vi "Stop cameras.vi"(4 "MASTER in":T1 {"Image data"."Color Palette" items=["Grayscale U8", "False Color", "Overexposed"]; "Image data"."Exposure time [us]" format="%#_10g"; "Queue"."Initial time [s]" format="%_19f"; "Queue"."Raw data [V]\n(all samples)" format="%0.2f"; "Queue"."Timestamp [s]" format="%_19f"}) -> ()   [LabVIEW 2020]
uses:
  MASTER.ctl
  Constants.ctl
  QBundle.ctl
  Queue.ctl
  Image data.ctl
  <vilib>/userdefined/High Color/IMAQdx.ctl
  <vilib>/vision/Image Controls.llb/IMAQ Image.ctl
  Image QBundle.ctl
  <vilib>/vision/driver/NI_Vision_Acquisition_Software.lvlib
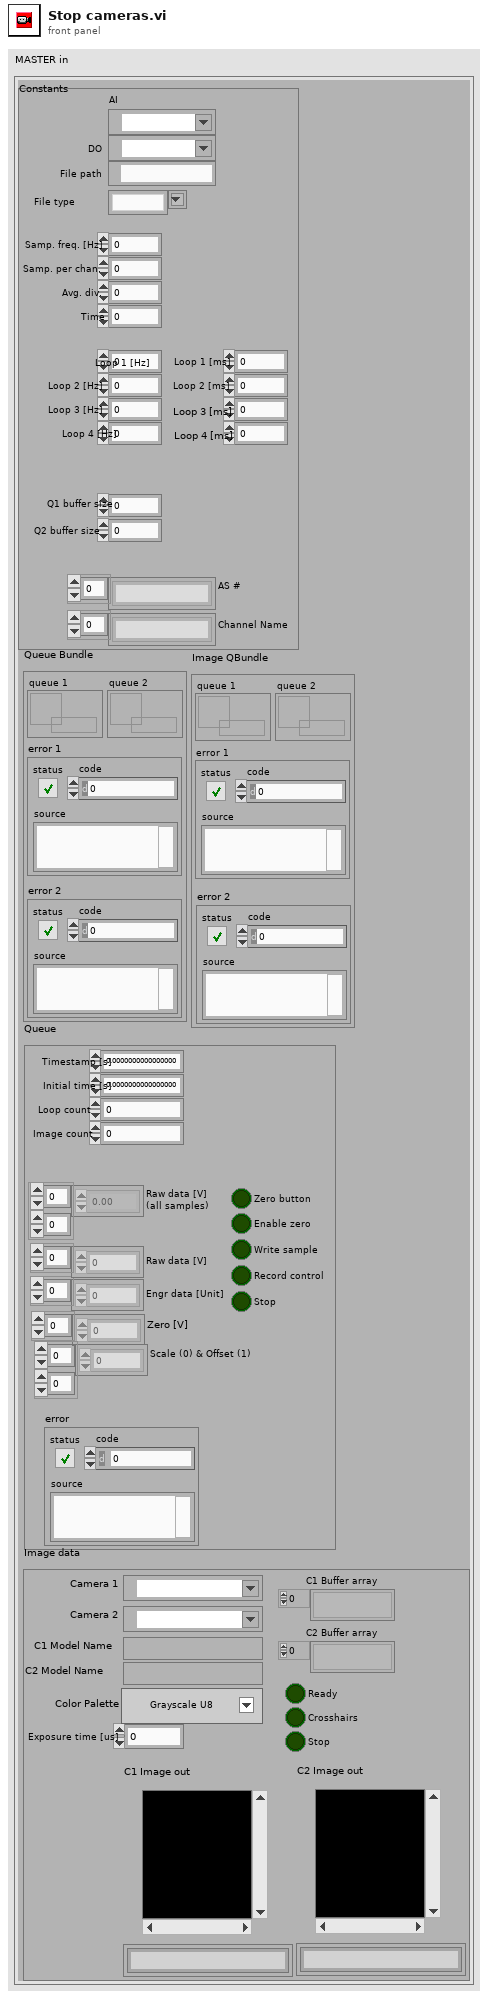
[diagram p1: front panel]
types:
  T1 = typedef "MASTER.ctl" = cluster{"Constants":T2, "Queue Bundle":T3, "Queue":T4, "Image data":T5, "Image QBundle ":T8}
  T2 = typedef "Constants.ctl" = cluster{"Time":u16, "Samp. freq. [Hz]":dbl, "Samp. per chan.":i32, "Avg. div.":i32, "File path":path, "AI":refnum<k21>, "Loop 1 [Hz]":dbl, "Loop 2 [Hz]":dbl, "Loop 3 [Hz]":dbl, "Loop 1 [ms]":dbl, "Loop 2 [ms]":dbl, "Loop 3 [ms]":dbl, "Q1 buffer size":i32, "Q2 buffer size":i32, "File type":string, "Loop 4 [Hz]":dbl, "Loop 4 [ms]":dbl, "Channel Name":string[], "AS #":string[], "DO":refnum<k21>}
  T3 = typedef "QBundle.ctl" = cluster{"queue 1":refnum<queue>, "error 1":errorcluster, "queue 2":refnum<queue>, "error 2":errorcluster}
  T4 = typedef "Queue.ctl" = cluster{"Enable zero":bool, "Engr data [Unit]":dbl[], "Zero button":bool, "Zero [V]":dbl[], "Timestamp [s]":dbl, "Write sample":bool, "Record control":bool, "Stop":bool, "error":errorcluster, "Raw data [V]\n(all samples)":dbl[][], "Raw data [V]":dbl[], "Loop count":i64, "Initial time [s]":dbl, "Scale (0) & Offset (1)":dbl[][], "Image count":dbl}
  T5 = typedef "Image data.ctl" = cluster{"Camera 1":T6, "Camera 2":T6, "C1 Image out ":T7, "C2 Image out":T7, "C1 Model Name":string, "C2 Model Name":string, "Exposure time [us]":dbl, "Color Palette":u16, "C1 Buffer array":T7[], "Ready":bool, "C2 Buffer array":T7[], "Crosshairs":bool, "Stop":bool}
  T6 = typedef "IMAQdx.ctl" = refnum<k21>
  T7 = typedef "IMAQ Image.ctl" = refnum<image>
  T8 = typedef "Image QBundle.ctl" = cluster{"queue 1":refnum<queue>, "error 1":errorcluster, "queue 2":refnum<queue>, "error 2":errorcluster}
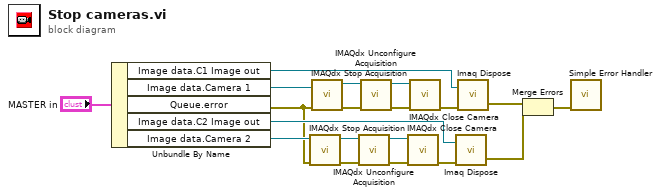
[diagram p0: block diagram]
diagram:
  n1 = Unbundle By Name("MASTER in") -> ("Image data.C1 Image out"=w12:T7, "Image data.Camera 1"=w15:T6, "Queue.error"=w6:errorcluster, "Image data.C2 Image out"=w7:T7, "Image data.Camera 2"=w8:T6)
  n2 = call <vilib>:"IMAQdx Stop Acquisition.vi"("error in"=w6, "Session In"=w8) -> ("error out"=w10:errorcluster, "Session Out"=w2:T6)  [unwired: 8 out]
  n3 = call <vilib>:"IMAQdx Stop Acquisition.vi"("error in"=w6, "Session In"=w15) -> ("error out"=w18:errorcluster, "Session Out"=w14:T6)  [unwired: 8 out]
  n4 = call <vilib>:"IMAQdx Unconfigure Acquisition.vi"("error in"=w10, "Session In"=w2) -> ("error out"=w11:errorcluster, "Session Out"=w1:T6)  [unwired: 8 out]
  n5 = call <vilib>:"IMAQdx Unconfigure Acquisition.vi"("error in"=w18, "Session In"=w14) -> ("error out"=w19:errorcluster, "Session Out"=w13:T6)  [unwired: 8 out]
  n6 = call <vilib>:"IMAQdx Close Camera.vi"("error in"=w11, "Session In"=w1) -> ("error out"=w9:errorcluster)  [unwired: 9 out]
  n7 = call <vilib>:"IMAQdx Close Camera.vi"("error in"=w19, "Session In"=w13) -> ("error out"=w17:errorcluster)  [unwired: 9 out]
  n8 = call "Imaq Dispose"("Image"=w7, "error in (no error)"=w9) -> ("error out"=w4:errorcluster)  [unwired: 4 in]
  n9 = call "Imaq Dispose"("Image"=w12, "error in (no error)"=w17) -> ("error out"=w3:errorcluster)  [unwired: 4 in]
  n10 = Merge Errors(w3, w4) -> (w5:errorcluster)
  n11 = call <vilib>:"Simple Error Handler.vi"("error in (no error)"=w5) -> ()  [unwired: 1 in, 8 out]
